vi "Queue.vi"() -> ()   [LabVIEW 2015]
panel:
  out "output variable":dbl
  in  "stop":bool
  in  "Numeric":i32
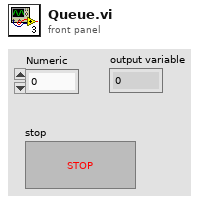
[diagram p1: front panel]
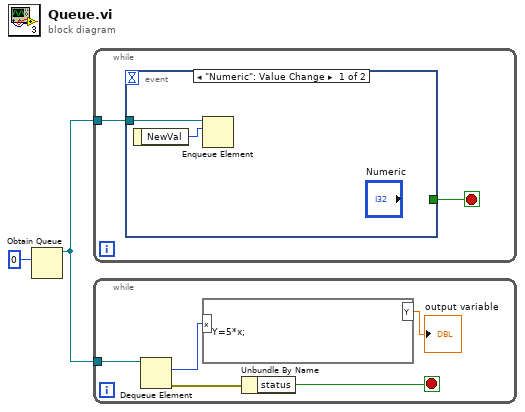
[diagram p0: block diagram]
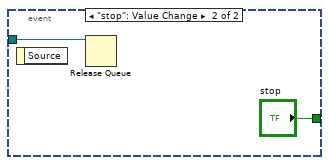
[diagram p2: hidden frame]
diagram:
  n1 = Obtain Queue(element data type=0) -> (queue out=w1:refnum<queue>)  [unwired: 4 in, 2 out]
  n2 = while {
    tunnel: w1 -> [w4]
    stop <- w3 stop-if-true
    n3 = event shown="[0] \"Numeric\": Value Change" {
      selector: _ -> [_ _]
      dyn-events: _ -> [_ _]
      timeout: _ -> [_ _]
      tunnel: w4 -> [w6 w8]
      tunnel: [_ "stop"] -> w3
      event "Numeric": Value Change {
        n4 = event-data() -> ("NewVal"=w5:i32)  [unwired: 1 in]
        n5 = Enqueue Element(queue=w6, element=w5) -> ()  [unwired: 2 in, 3 out]
      }
      event "stop": Value Change {
        n6 = event-data() -> ()  [unwired: 1 in, 1 out]
        n7 = Release Queue(queue=w8) -> ()  [unwired: 2 in, 3 out]
      }
    }
  }
  n8 = while {
    tunnel: w1 -> [w13]
    stop <- w9 stop-if-true
    n9 = Dequeue Element(queue=w13) -> (element=w12:i32, error out=w10:errorcluster)  [unwired: 2 in, 2 out]
    n10 = formula code="Y=5*x;"("x"=w12) -> ("Y"=→"output variable":dbl)
    n11 = Unbundle By Name(w10) -> ("status"=w9:bool)
  }
